vi "Actor Core.vi"(8 "error in":errorcluster caption="错误输入", 11 "UI in":refnum<class "UI.lvclass"> caption="操作者输入") -> (0 "error out":errorcluster caption="错误输出", 3 "Actor out":refnum<class "Actor.lvclass"> caption="操作者输出")   [LabVIEW 2018, in "UI.lvlib" / "UI.lvclass"]
doc: "(<B>文件名</B>: Actor Framework.lvlib:Actor.lvclass:Actor Core.vi)\n\n接收发送至操作者的消息，响应消息并处理可能导致操作者关闭的错误。\n\n子孙类重写该VI，使操作者完成特定的任务。使用调用父方法节点实现重写。"
uses:
  UI.lvclass
  <vilib>/ActorFramework/Actor/Actor.lvclass
panel:
  in  "确定按钮":bool
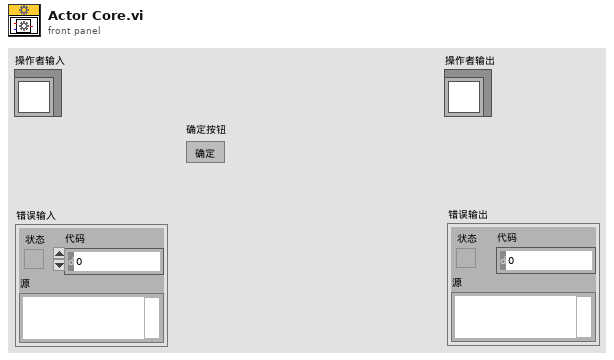
[diagram p1: front panel]
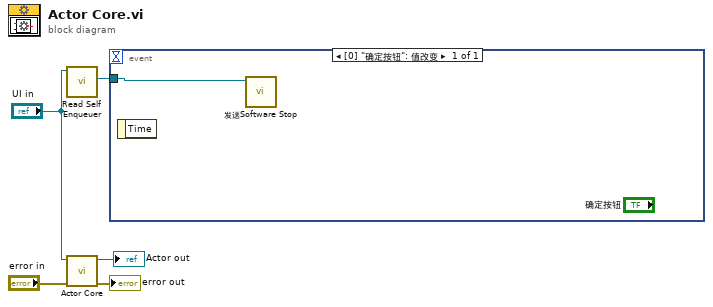
[diagram p0: block diagram]
diagram:
  n1 = call <vilib>:"Read Self Enqueuer.vi"("Actor"="UI in") -> ("Self Enqueuer"=w2:refnum<class "Message Enqueuer.lvclass">)  [unwired: 10 in]
  n2 = call-parent "Actor Core.vi"("error in"="error in", "Actor in"="UI in") -> ("error out"=→"error out":errorcluster, "Actor out"=→"Actor out":refnum<class "Actor.lvclass">)  [unwired: 8 in]
  n3 = event shown="[0] \"确定按钮\": 值改变" {
    selector: _ -> [_]
    dyn-events: _ -> [_]
    timeout: _ -> [_]
    tunnel: w2 -> [w6]
    event "确定按钮": Value Change {
      n4 = event-data() -> ()  [unwired: 1 in, 1 out]
      n5 = call "发送Software Stop.vi"("Message Enqueuer"=w6) -> ()  [unwired: 9 in, 2 out]
    }
  }
